vi "Cmd - Build.vi"(8 "error in (no error)":errorcluster, 11 "NIPKG Packager in":refnum<class "NIPKG Packager.lvclass">) -> (0 "error out":errorcluster, 3 "NIPKG Packager out":refnum<class "NIPKG Packager.lvclass">)   [LabVIEW 2019, in "NIPKG Packager.lvclass"]
uses:
  NIPKG Packager.lvclass
  NIPKG Packager.lvclass/NIPKG Packager.ctl
  CLI Output/CLI Output.lvclass
panel:
  out "standard error":string
  out "standard output":string
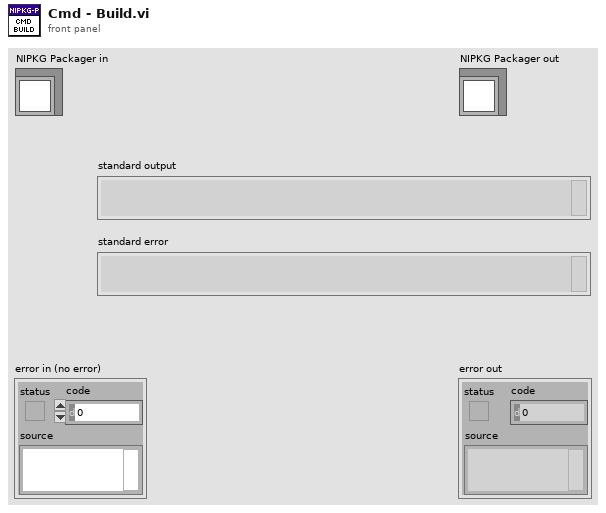
[diagram p1: front panel]
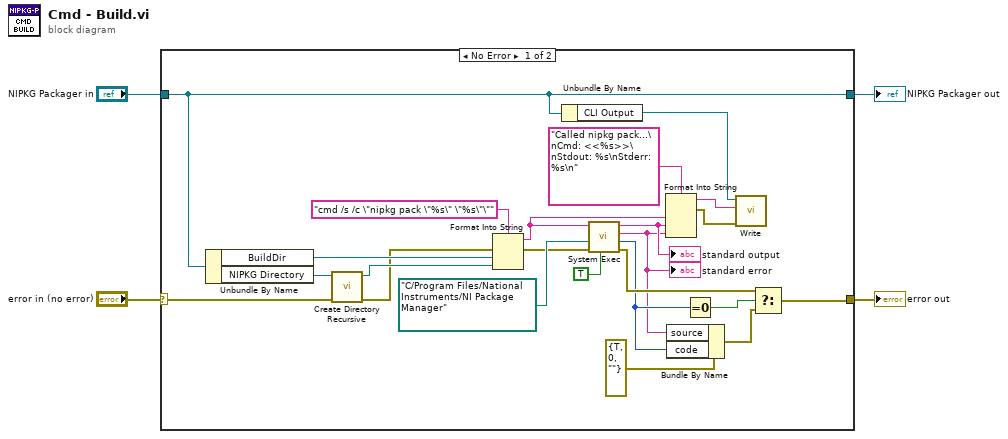
[diagram p0: block diagram]
diagram:
  n1 = case shown="No Error" "error in (no error)" {
    selector: "error in (no error)" -> [w21 w29]
    tunnel: [w9 w29] -> w3
    tunnel: [w19 w28] -> w1
    tunnel: "NIPKG Packager in" -> [w19 w28]
    frame No Error {
      n2 = Unbundle By Name(w19) -> ("BuildDir"=w24:path, "NIPKG Directory"=w23:path)
      n3 = call <vilib>:"Create Directory Recursive.vi"("error in (no error)"=w21, "directory"=w23) -> ("error out"=w20:errorcluster, "directory copy"=w22:path)  [unwired: 3 in, 1 out]
      n4 = Format Into String(format string="cmd /s /c \"nipkg pack \"%s\" \"%s\"\"", error in=w20, w24, w22) -> (resulting string=w12:string, error out=w25:errorcluster)  [unwired: 1 in]
      n5 = Unbundle By Name(w19) -> ("CLI Output"=w17:refnum<class "CLI Output.lvclass">)
      n6 = call <vilib>:"System Exec.vi"("run minimized? (F)"=TRUE, "error in (no error)"=w25, "working directory"=path "C:/Program Files/National Instruments/NI Package Manager", "command line"=w12) -> ("error out"=w10:errorcluster, "return code"=w6:i32, "standard error"=w5:string, "standard output"=w18:string)  [unwired: 4 in]
      "standard output" <- w18
      "standard error" <- w5
      n7 = Format Into String(format string="Called nipkg pack...\nCmd: <<%s>>\nStdout: %s\nStderr: %s\n", w12, w18, w5) -> (resulting string=w16:string, error out=w15:errorcluster)  [unwired: 2 in]
      n8 = Bundle By Name(cluster=errorcluster {"status"=TRUE, "code"=0, "source"=""} ("error constant"), "source"=w5, "code"=w6) -> (w7:errorcluster)
      n9 = Equal To 0?(x=w6) -> (x = 0?=w11:bool)
      n10 = call-dynamic "Write.vi"("error in (no error)"=w15, "String"=w16, "CLI Output in"=w17) -> ()  [unwired: 7 in, 2 out]
      n11 = Select(t=w10, s=w11, f=w7) -> (s? t:f=w9:errorcluster)
    }
    frame Error {
    }
  }
  "error out" <- w3
  "NIPKG Packager out" <- w1
